vi "类信息.vi"() -> ()   [LabVIEW 2014]
uses:
  RT/utils_RT/cRIO Convert Thermocouple Readings.llb/Thermocouple Type.ctl
panel:
  in  "0_模块注册消息类":T1={"标题"="未命名", "相对路径"="R\\activity模板.vi", "类型"=enum."活动", "专属队列名称"="yQPC7c1ByUa59utYbVeowZ9iPz3wrH"}
  in  "0_消息类":cluster{"消息":string, "数据":variant}
  in  "主界面配置类":T2={"侧边栏数据"=[], "界面刷间隔率"=1000.0}
  in  "热电偶参数类":cluster{"型号":T3}={"型号"=2} {"型号" items=["B", "E", "J", "K", "R", "S", "T", "N"]}
  in  "热电阻参数簇":cluster{"A":dbl, "B":dbl, "C":dbl}
  in  "compactRIO配置类":T4
  in  "板卡信息类":T5
  in  "索引数据类":cluster{"来源":string, "名称":string}
  in  "show配置类":T6
  in  "串口配置类":T7={"串口资源名称"="", "波特率"=9600, "数据比特"=8, "奇偶"=0, "停止位"=15, "流控制"=0, "超时"=10000}
  in  "数据属性类":T8
  in  "应用信息类":T9
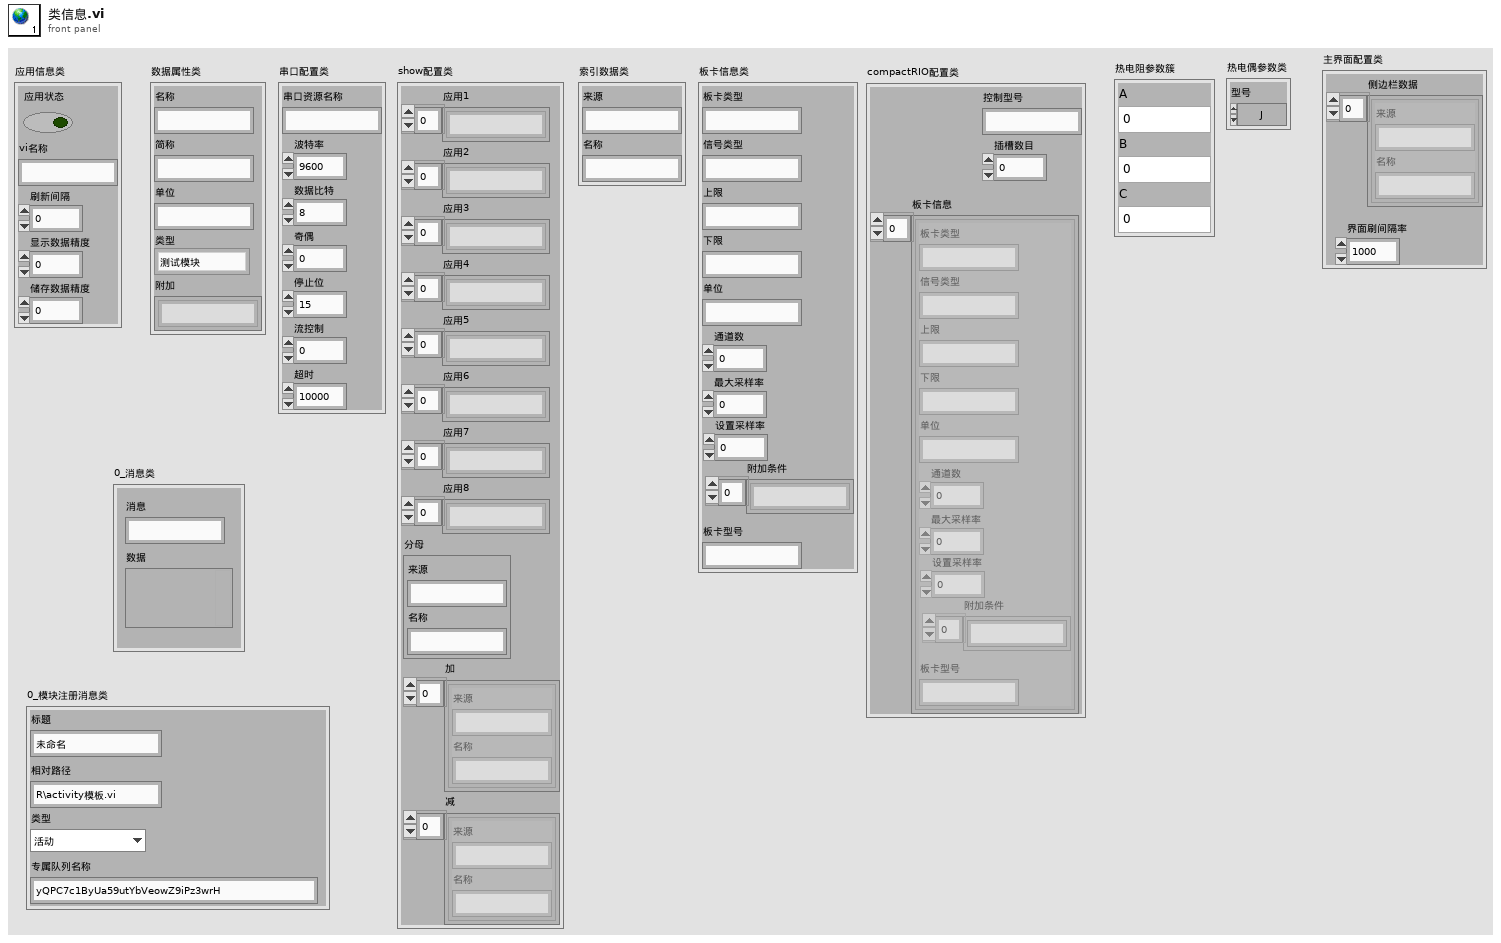
[diagram p1: front panel]
types:
  T1 = cluster{"标题":string, "相对路径":string, "类型":enum16{"服务", "活动"}, "专属队列名称":string}
  T2 = cluster{"侧边栏数据":cluster{"来源":string, "名称":string}[], "界面刷间隔率":dbl}
  T3 = typedef "Thermocouple Type.ctl" = u16
  T4 = cluster{"控制型号":string, "插槽数目":u32, "板卡信息":cluster{"板卡类型":string, "信号类型":string, "上限":string, "下限":string, "单位":string, "通道数":u32, "最大采样率":u32, "设置采样率":u32, "附加条件":string[], "板卡型号":string}[]}
  T5 = cluster{"板卡类型":string, "信号类型":string, "上限":string, "下限":string, "单位":string, "通道数":u32, "最大采样率":u32, "设置采样率":u32, "附加条件":string[], "板卡型号":string}
  T6 = cluster{"应用1":string[], "应用2":string[], "应用3":string[], "应用4":string[], "应用5":string[], "应用6":string[], "应用7":string[], "应用8":string[], "分母":cluster{"来源":string, "名称":string}, "加":cluster{"来源":string, "名称":string}[], "减":cluster{"来源":string, "名称":string}[]}
  T7 = cluster{"串口资源名称":string, "波特率":u32, "数据比特":u32, "奇偶":u32, "停止位":u32, "流控制":u32, "超时":u32}
  T8 = cluster{"名称":string, "简称":string, "单位":string, "附加":string[], "类型":enum16{"测试模块", "FPGA", "cRIO", "其他设备", "总体展示"}}
  T9 = cluster{"应用状态":bool, "vi名称":string, "刷新间隔":u32, "显示数据精度":u32, "储存数据精度":u32}
diagram:
